vi "glb_source.vi"() -> ()   [LabVIEW 2014]
panel:
  in  "循环计数":i32
  in  "112箱内灯":bool
  in  "111灯带4":bool
  in  "110灯带3":bool
  in  "109灯带2":bool
  in  "108灯带1":bool
  in  "107玻璃变色":bool
  in  "106复位":bool
  in  "105体验结束":bool
  in  "104开始体验":bool
  in  "103开门":bool
  in  "102急停状态":bool
  in  "stop":bool
  in  "URI_更新设备状态":string="https://tst-api-iot.uaes.com/cessshow/v1/device/status?status="
  in  "URI_请求命令参数":string="https://tst-api-iot.uaes.com/cessshow/v1/cmd/get?deviceId=ces_device_1"
  in  "URI_结束视频":string="source\\test3.mov"
  in  "URI_体验视频":string="source\\test2.mov"
  in  "URI_欢迎视频":string="source\\test1.mp4"
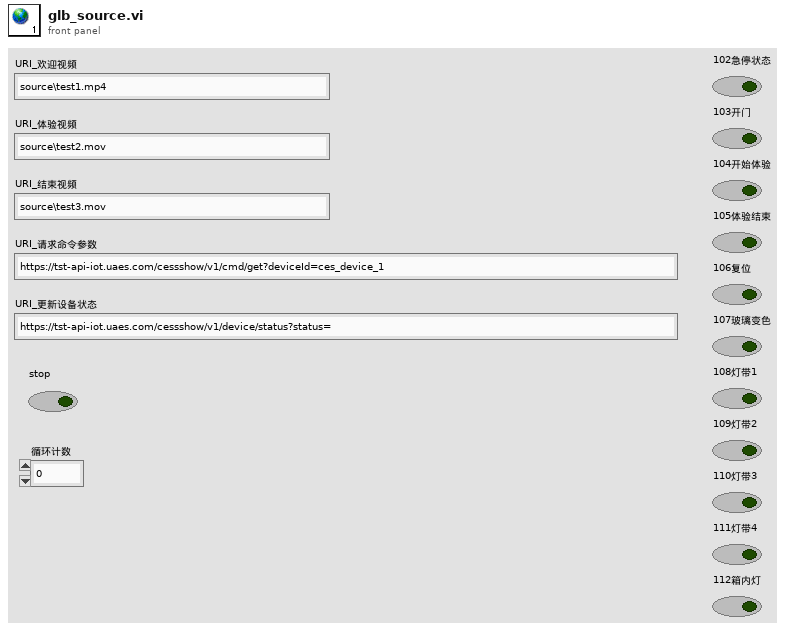
[diagram p1: front panel]
diagram:
